vi "Change Oven Type.vi"(8 "error in (no error)":errorcluster, 10 "New Oven Type":refnum<class "Oven Actor.lvclass">, 11 "Oven Actor in":refnum<class "Oven Actor.lvclass">) -> (0 "error out":errorcluster, 3 "Oven Actor out":refnum<class "Oven Actor.lvclass">)   [LabVIEW 2024, in "Oven Actor.lvlib" / "Oven Actor.lvclass"]
uses:
  Oven Actor.lvclass
  Oven Actor.lvclass/Oven Actor.ctl
  C:/Program Files/National Instruments/LabVIEW 2024/vi.lib/ActorFramework/Actor/Actor.lvclass
  C:/Users/burakkorkmaz/Desktop/Leveling/repo/Oven Actor/Oven Actor/Oven Actor.lvclass
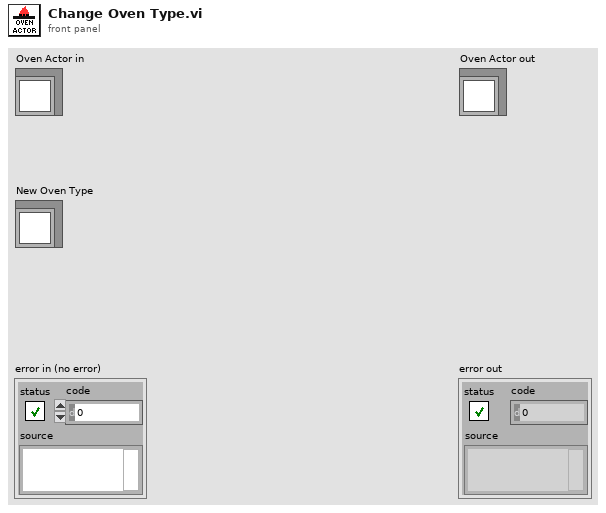
[diagram p1: front panel]
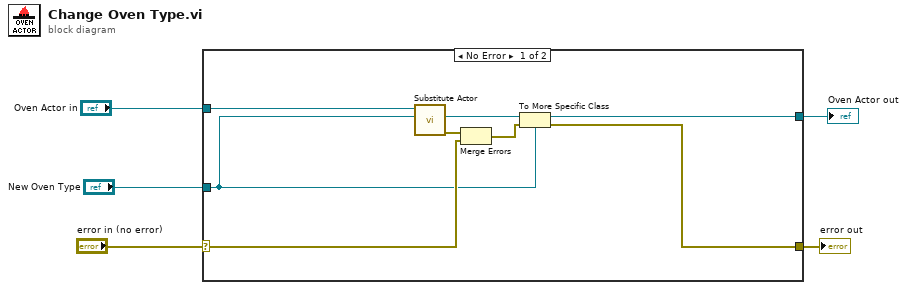
[diagram p0: block diagram]
diagram:
  n1 = case shown="No Error" "error in (no error)" {
    selector: "error in (no error)" -> [w12 w15]
    tunnel: [w11 w15] -> w4
    tunnel: [w6 w14] -> w2
    tunnel: "Oven Actor in" -> [w13 w14]
    tunnel: "New Oven Type" -> [w7 _]
    frame No Error {
      n2 = call-dynamic "Substitute Actor.vi"("Substitute Actor in"=w7, "Current Oven Actor"=w13) -> ("error out"=w9:errorcluster, "Substitute Actor out"=w8:refnum<class "Actor.lvclass">)  [unwired: 8 in]
      n3 = Merge Errors(w9, w12) -> (w10:errorcluster)
      n4 = To More Specific Class(target class=w7, reference=w8, error in=w10) -> (specific class reference=w6:refnum<class "Oven Actor.lvclass">, error out=w11:errorcluster)
    }
    frame Error {
    }
  }
  "error out" <- w4
  "Oven Actor out" <- w2
